vi "LoadVI.vi"(0 "LabVIEW In":refnum<vi>, 1 "Address":string="localhost", 2 "Path":path, 3 "Options":i32=16 format="%.0x", 4 "Port":u16=3364, 5 "Name":string, 7 "Type":refnum<vi>) -> (6 "LabVIEW Out":refnum<vi>, 8 "Reference":refnum<vi>)   [LabVIEW 2014]
uses:
  LabVIEW.vi
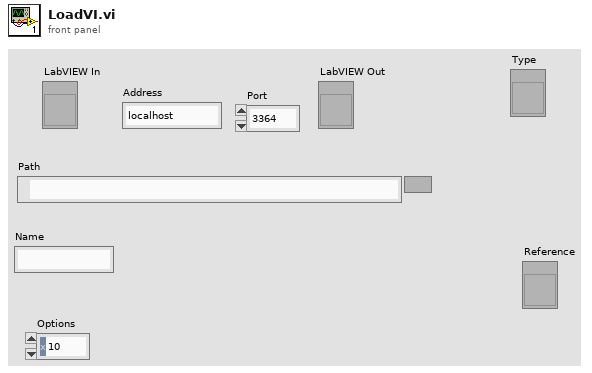
[diagram p1: front panel]
types:
  T1 = cluster{"Name":string, "Reference":refnum<vi>, "Ctrls":cluster{"Name":string, "Ctrl":refnum<vi>}[]}
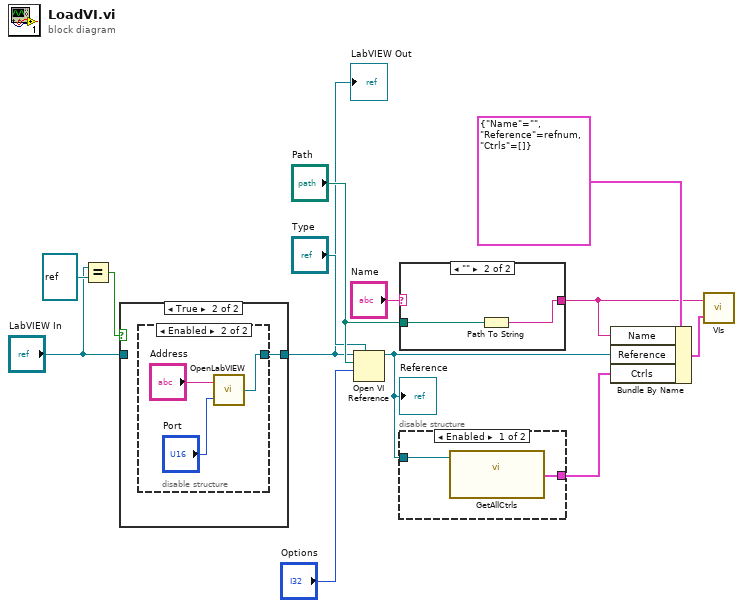
[diagram p0: block diagram]
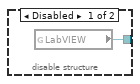
[diagram p3: hidden frame]
diagram:
  n1 = Equal?(x="LabVIEW In", y=refnum<vi> refnum ("LabVIEW")) -> (x = y?=w3:bool)
  n2 = case shown="True" w3 {
    tunnel: [w14 w15] -> w1
    tunnel: "LabVIEW In" -> [w14 _]
    frame False {
    }
    frame True {
      n3 = disable-structure shown="Enabled" {
        disable-tunnel: [w16 w17] -> w15
        frame Disabled {
          n4 = global read "LabVIEW.vi" "LabVIEW"() -> (w16:refnum<vi>)
        }
        frame Enabled {
          n5 = call "OpenLabVIEW.vi"("Port"="Port", "Address"="Address") -> ("LabVIEW"=w17:refnum<vi>)
        }
      }
    }
  }
  "LabVIEW Out" <- w1
  n6 = Open VI Reference(type specifier VI Refnum (for type only)="Type", application reference (local)=w1, vi path="Path", options="Options") -> (vi reference=w11:refnum<vi>)  [unwired: 2 in, 1 out]
  "Reference" <- w11
  n7 = case shown="\"\"" "Name" {
    selector: "Name" -> [w20 _]
    tunnel: "Path" -> [_ w22]
    tunnel: [w20 w21] -> w6
    frame Default {
    }
    frame "" {
      n8 = Path To String(path=w22) -> (string=w21:string)
    }
  }
  n9 = disable-structure shown="Enabled" {
    disable-tunnel: w11 -> [w24 _]
    disable-tunnel: [w23 _] -> w10
    frame Enabled {
      n10 = call "GetAllCtrls.vi"("VI"=w24) -> ("Ctrls"=w23:cluster{"Name":string, "Ctrl":refnum<vi>}[])  [unwired: 1 in]
    }
    frame Disabled {
    }
  }
  n11 = Bundle By Name(cluster=T1 {"Name"="", "Reference"=refnum, "Ctrls"=[]} ("VI In"), "Name"=w6, "Reference"=w11, "Ctrls"=w10) -> (w9:T1)
  n12 = call "VIs.vi"("VI In"=w9, "Name"=w6) -> ()  [unwired: 1 out]
